vi "UART Write Data.vi"(7 "UART #":T1=-1, 8 "error in (no error)":errorcluster, 10 "Data":string, 11 "Session in":refnum<class "Session.lvclass">) -> (0 "error out":errorcluster, 3 "Session out":refnum<class "Session.lvclass">)   [LabVIEW 2020, in "CTI.lvlib" / "Session.lvclass"]
uses:
  Session.lvclass
  UART Number.ctl
  DeviceComms/DeviceComms.lvclass
  CTI.lvlib
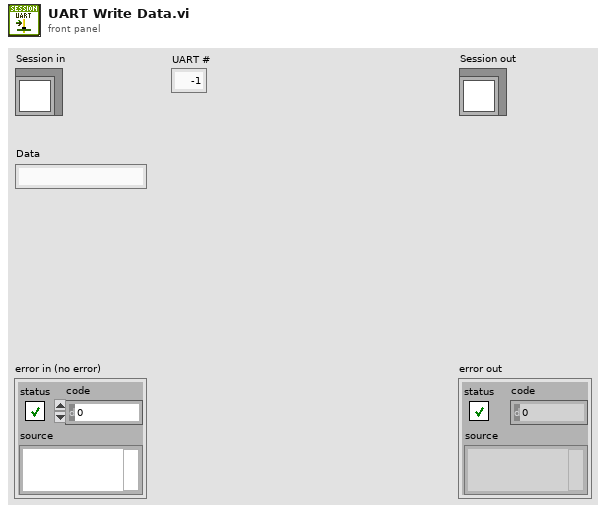
[diagram p1: front panel]
types:
  T1 = typedef "CTI.lvlib/UART Number.ctl" = i8
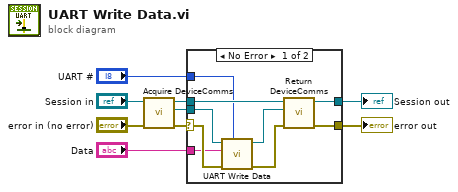
[diagram p0: block diagram]
diagram:
  n1 = call "Acquire DeviceComms.vi"("error in (no error)"="error in (no error)", "Session in"="Session in") -> ("error out"=w8:errorcluster, "DeviceComms"=w7:refnum<class "DeviceComms.lvclass">, "Session out"=w9:refnum<class "Session.lvclass">)  [unwired: 7 in]
  n2 = case shown="No Error" w8 {
    selector: w8 -> [w17 w20]
    tunnel: w9 -> [w16 w19]
    tunnel: w7 -> [w18 _]
    tunnel: [w13 w19] -> w2
    tunnel: [w12 w20] -> w1
    tunnel: "UART #" -> [w11 _]
    tunnel: "Data" -> [w10 _]
    frame No Error {
      n3 = call-dynamic "UART Write Data.vi"("UART #"=w11, "error in (no error)"=w17, "Data"=w10, "DeviceComms in"=w18) -> ("error out"=w14:errorcluster, "DeviceComms out"=w15:refnum<class "DeviceComms.lvclass">)  [unwired: 6 in]
      n4 = call "Return DeviceComms.vi"("error in (no error)"=w14, "DeviceComms"=w15, "Session in"=w16) -> ("error out"=w12:errorcluster, "Session out"=w13:refnum<class "Session.lvclass">)  [unwired: 7 in]
    }
    frame Error {
    }
  }
  "error out" <- w1
  "Session out" <- w2
